vi "P11_Sequence.vi"() -> ()   [LabVIEW 2022 SP3]
panel:
  in  "Slide":dbl(slide) scale=1.0..1000.0
  out "Numeric":dbl
  in  "stop":bool
  in  "Boolean 5":bool
  out "Boolean 4":bool
  out "Boolean 3":bool
  out "Boolean 2":bool
  out "Boolean":bool
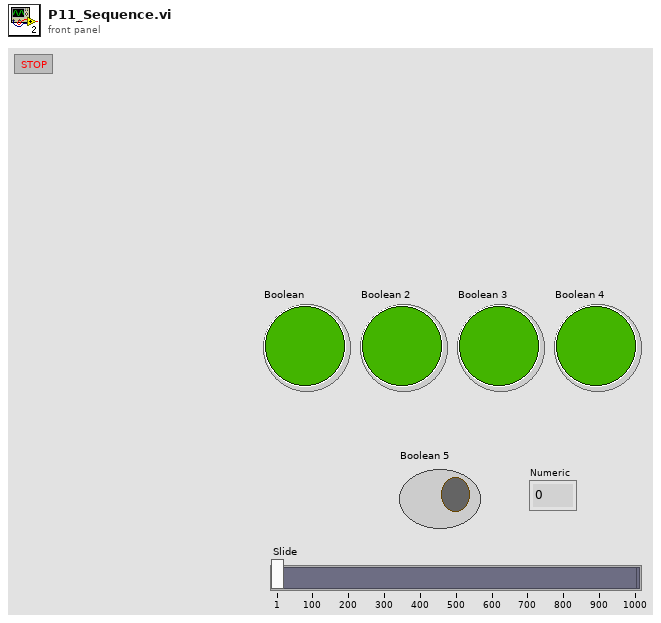
[diagram p1: front panel]
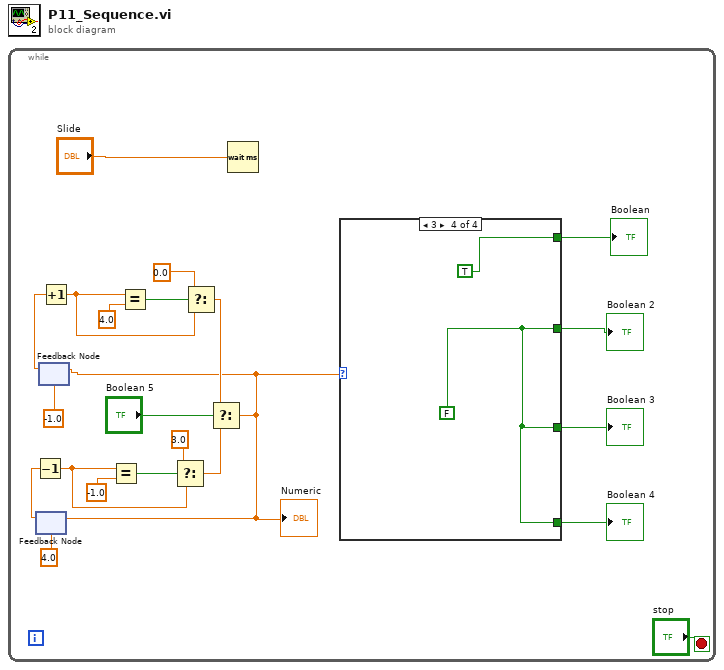
[diagram p0: block diagram]
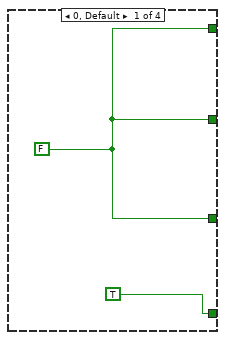
[diagram p2: hidden frame]
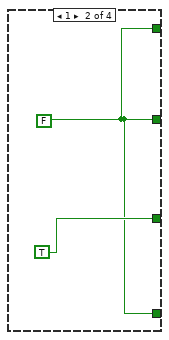
[diagram p3: hidden frame]
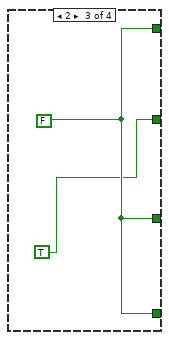
[diagram p4: hidden frame]
diagram:
  n1 = while {
    stop <- "stop" stop-if-true
    n2 = feedback #1(4.0) -> (w14:dbl)
    n3 = Decrement(x=w14) -> (x-1=w9:dbl)
    n4 = feedback #2(-1.0) -> (w21:dbl)
    n5 = Increment(x=w21) -> (x+1=w17:dbl)
    n6 = Equal?(x=w9, y=-1.0) -> (x = y?=w11:bool)
    n7 = Equal?(x=w17, y=4.0 ("x")) -> (x = y?=w19:bool)
    n8 = Select(t=3.0, s=w11, f=w9) -> (s? t:f=w7:dbl)
    n9 = Select(t=0.0, s=w19, f=w17) -> (s? t:f=w8:dbl)
    n10 = Select(t=w8, s="Boolean 5", f=w7) -> (s? t:f=w5:dbl)
    "Numeric" <- w5
    n11 = feedback-in #1(w5) -> ()
    n12 = feedback-in #2(w5) -> ()
    n13 = Wait (ms)(milliseconds to wait="Slide") -> ()  [unwired: 1 out]
    n14 = case shown="3" w5 {
      tunnel: [w24 w25 w28 TRUE] -> w4
      tunnel: [w24 w25 TRUE w29] -> w3
      tunnel: [w24 TRUE w28 w29] -> w2
      tunnel: [TRUE w25 w28 w29] -> w1
      frame 0, Default {
        w24 = FALSE
      }
      frame 1 {
        w25 = FALSE
      }
      frame 2 {
        w28 = FALSE
      }
      frame 3 {
        w29 = FALSE
      }
    }
    "Boolean" <- w4
    "Boolean 2" <- w3
    "Boolean 3" <- w2
    "Boolean 4" <- w1
  }
